vi "GetImpModeStr.vi"(8 "错误输入（无错误）":errorcluster, 9 "阻抗模式索引":u8, 10 "字符串分配空间大小":u32, 11 "阻抗模式描述":string) -> (0 "错误输出":errorcluster, 3 "阻抗模式描述":string)   [LabVIEW 2014]
uses:
  X86Dll/ZXUTConfigMgr.dll
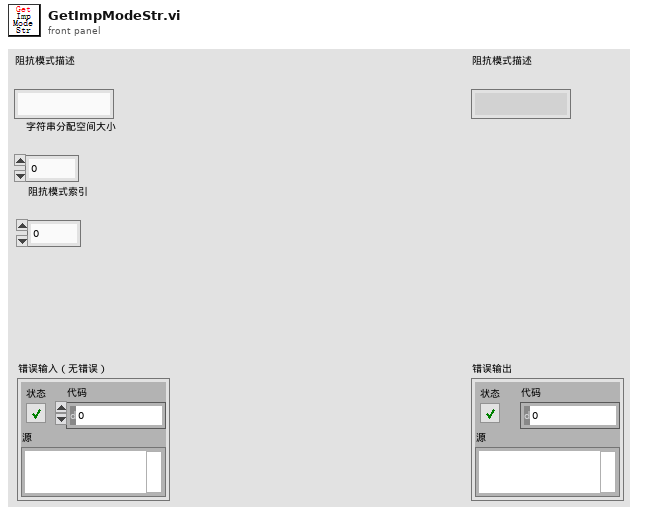
[diagram p1: front panel]
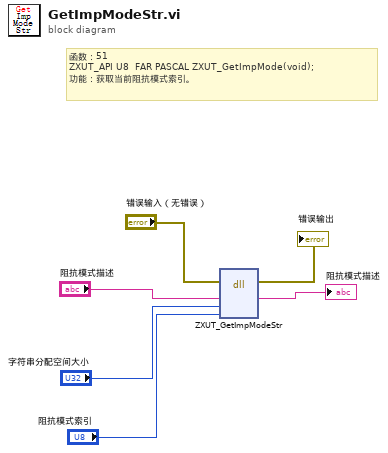
[diagram p0: block diagram]
diagram:
  # "函数：51\nZXUT_API U8\t\tFAR PASCAL ZXUT_GetImpMode(void);\n功能：获取当前阻抗模式索引。"
  n1 = dll-call lib="D:/Software/Utrasonic on-line monitoring/X86Dll/ZXUTConfigMgr.dll" fn="ZXUT_GetImpModeStr"(error in="错误输入（无错误）", "str"="阻抗模式描述", "nStrSize"="字符串分配空间大小", "Mode"="阻抗模式索引") -> (error out=→"错误输出":errorcluster, "str"=→"阻抗模式描述":string)  [unwired: 5 in, 1 out]
